vi "myRIO_BRig_FPGA_v3,1__PortC.vi"() -> ()   [LabVIEW 2014]
uses:
  <vilib>/rvi/FXPMathLib/FxpDiv/subVIs/nifxpmath_Div_SimConfig.ctl
  <vilib>/rvi/FXPMathLib/FxpSinAndCos/subVIs/nifxpmath_SinAndCos_SimConfig.ctl
  <vilib>/rvi/FXPMathLib/FxpDiv/simVIs/DllFxpDivTemp_sub.vi
  <vilib>/rvi/FXPMathLib/FxpSinAndCos/simVIs/DllFxpSinAndCosTemp_sub.vi
  <vilib>/rvi/Emulation/niFpgaGetClockAttributes.vi
  <vilib>/rvi/Emulation/niFpgaSctlEmulationGetInTimedLoop.vi
  <vilib>/rvi/Emulation/niFpgaEmulationReportErrorSimple.vi
  <vilib>/rvi/eio/common/nirviEmuTemplateMethod_errors.vi
  <vilib>/rvi/Emulation/niFpgaCriticalErrorInLSC.vi
  <vilib>/rvi/FXPMathLib/FxpDiv/XNode/nifxpmath_Div.xnode
  <vilib>/rvi/FXPMathLib/FxpMul/XNode/nifxpmath_Multiplier.xnode
  <vilib>/rvi/FXPMathLib/FxpSinAndCos/XNode/nifxpmath_SinAndCos.xnode
  <vilib>/rvi/FXPMathLib/FxpSub/XNode/nifxpmath_Sub.xnode
  <vilib>/eio/EIONode/EIONode.xnode
  <vilib>/rvi/FXPMathLib/sim/FxpSim.dll
panel:
  in  "AO0":i16
  in  "f_time_select":u32=173
  in  "laser_Nvalley":u32=100
  in  "laser_Npeak":u32=100
  in  "laserledMTrig":bool
  in  "tCycle_laser_wro":u32=100
  in  "tDelay_laser_wro":u32
  in  "tCycle_laser_rew":u32=100
  in  "tDelay_laser_rew":u32
  in  "laserResponse_reward_LED":bool
  in  "laserResponse_wrong_LED":bool
  out "SelectWrong":bool
  out "SelectReward":bool
  in  "laserResponse_wrong":bool
  in  "laserResponse_reward":bool
  in  "Left(F)_or_Right(T)":bool
  in  "ignoreWrong":bool
  in  "SelectionState":bool
  in  "laserMTrig":bool
  in  "FPGA_Stop":bool
  in  "audioTrigger_L":bool
  in  "audioTrigger_R":bool
  in  "audioFreq_L_Hz":u16=1000 min=1000 max=14000 step=1000
  in  "audioAmp_L":u16=1 min=1 max=32767 step=1
  in  "audioFreq_R_Hz":u16=1000 min=1000 max=14000 step=1000
  in  "audioAmp_R":u16=1 min=1 max=32767 step=1
  in  "A3_SL":bool
  in  "A1_SR":bool
  in  "Counts_Reset":bool
  out "A4_LickR":u32
  out "A2_LickL":u32
  in  "A6_Act":bool
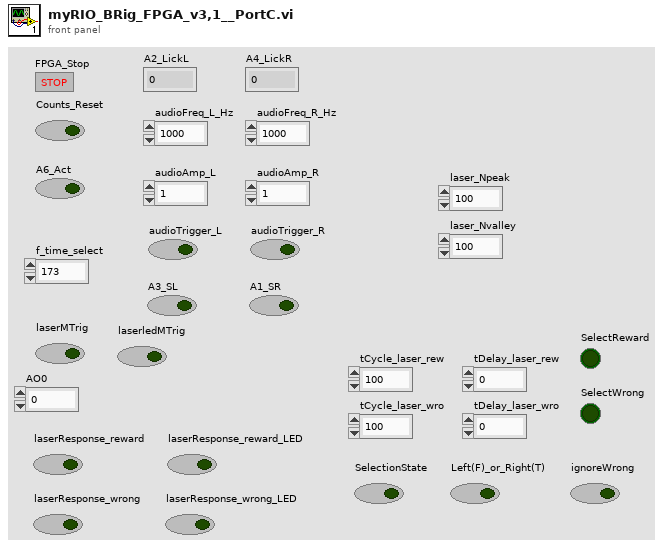
[diagram p1: front panel]
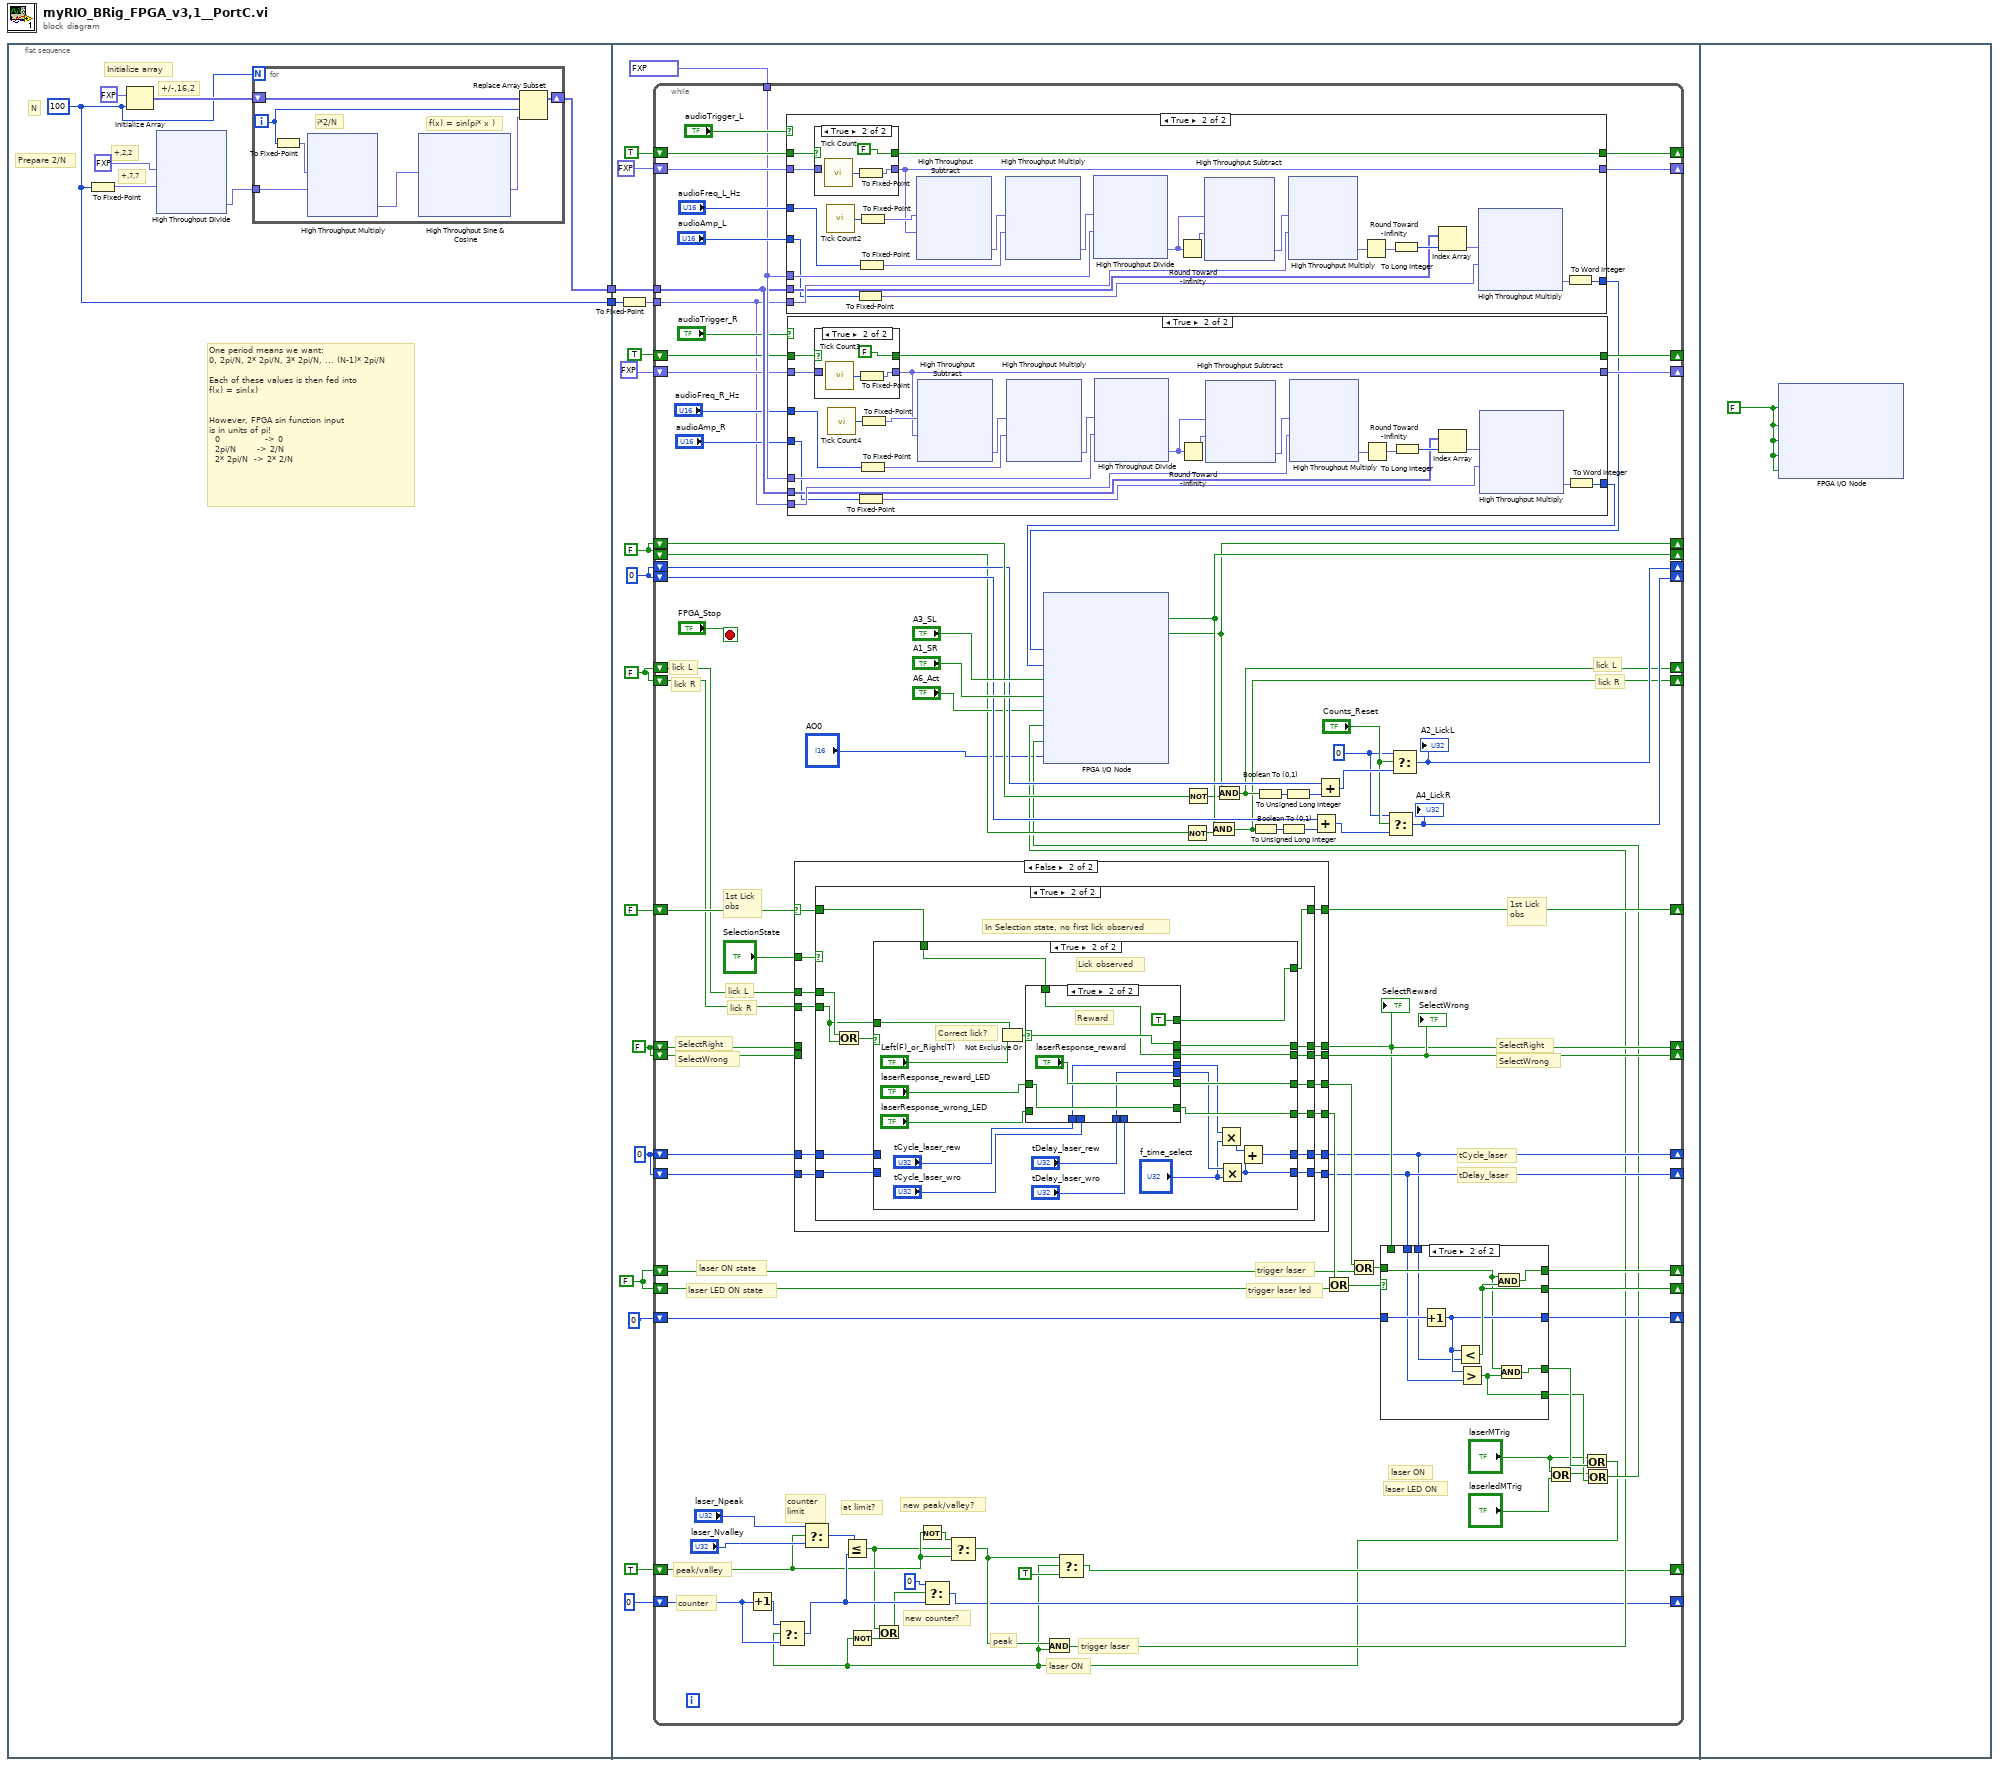
[diagram p0: block diagram]
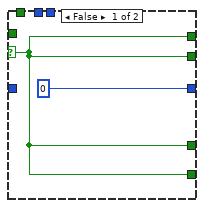
[diagram p2: hidden frame]
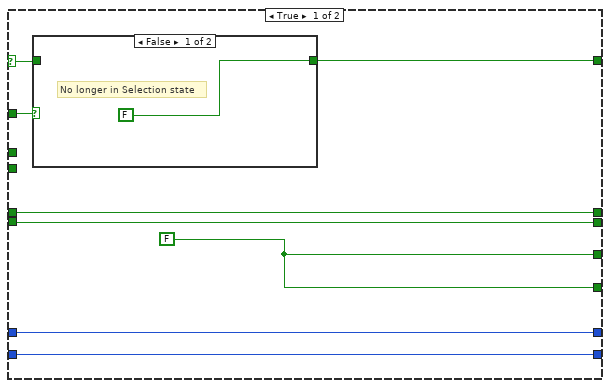
[diagram p3: hidden frame]
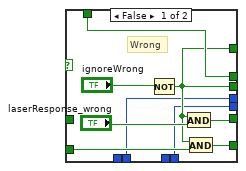
[diagram p7: hidden frame]
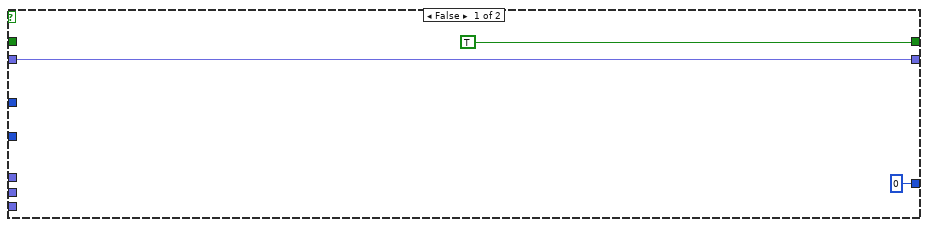
[diagram p8: hidden frame]
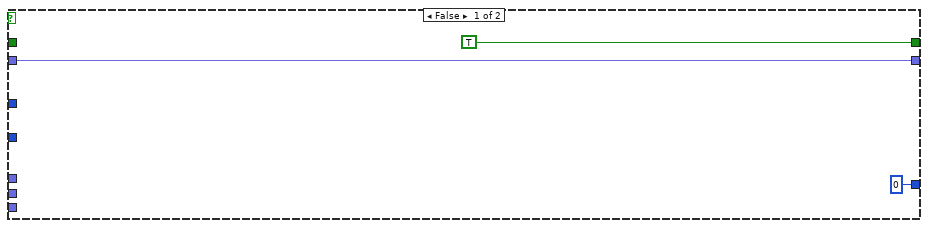
[diagram p10: hidden frame]
diagram:
  n1 = flat-sequence {
    tunnel: [w4] -> w2
    tunnel: [w3] -> w1
    tunnel: w2 -> [w86]
    tunnel: w1 -> [w88]
    frame #0 {
      w3 = 100 ("dimension size")
      # "N"
      # "+,7,7"
      # "+,2,2"
      # "+/-,16,2"
      # "Prepare 2/N"
      # "One period means we want:\n0, 2pi/N, 2* 2pi/N, 3* 2pi/N, ... (N-1)* 2pi/N\n\nEach of these values is then fed into\nf(x) = sin(x)\n\n\nHowever, FPGA sin function input\nis in units of pi!\n  0               -> 0\n  2pi/N       -> 2/N\n  2* 2pi/N  -> 2* 2/N"
      # "Initialize array"
      n2 = To Fixed-Point(number=w3) -> (fixed-point=w6:fxp<+,7,7>)  [unwired: 1 in]
      n3 = Initialize Array(fxp<+/-,16,2> 0.0 ("element"), w3) -> (w9:fxp<+/-,16,2>[])
      n4 = xnode "High Throughput Divide"("x"=fxp<+,2,2> 2.0, "y"=w6) -> ("x/y"=w5:fxp<+,27,0>)
      n5 = for {
        N: w3 -> [_]
        shift-right: [w42] -> w4
        shift-left: w9 -> [w43]
        tunnel: w5 -> [w38]
        i -> [w41]
        # "f(x) = sin(pi* x )"
        # "i*2/N"
        n6 = To Fixed-Point(number=w41) -> (fixed-point=w39:fxp<+,7,7>)  [unwired: 1 in]
        n7 = xnode ("High Throughput Multiply")("x"=w39, "y"=w38) -> ("x*y"=w37:fxp<+,34,7>)
        n8 = xnode "High Throughput Sine & Cosine"("x (pi)"=w37) -> ("sin(x)"=w40:fxp<+/-,16,2>)  [unwired: 1 out]
        n9 = Replace Array Subset(array=w43, new element=w40, index=w41) -> (w42:fxp<+/-,16,2>[])
      }
    }
    frame #1 {
      w76 = u32 0
      w78 = FALSE
      w77 = FALSE
      w81 = FALSE
      w82 = FALSE
      w83 = u32 0
      n10 = To Fixed-Point(number=w88) -> (fixed-point=w87:fxp<+,7,7>)  [unwired: 1 in]
      n11 = while {
        shift-right: [w176] -> _
        shift-left: TRUE -> [w180]
        shift-right: [w175] -> _
        shift-left: fxp<+,32,32> 0.0 -> [w179]
        tunnel: fxp<+,17,26> 40000000.0 -> [w174]
        tunnel: w87 -> [w167]
        tunnel: w86 -> [w173]
        shift-right: [w166] -> _
        shift-left: TRUE -> [w172]
        shift-right: [w165] -> _
        shift-left: fxp<+,32,32> 0.0 -> [w171]
        shift-right: [w142] -> _
        shift-left: w83 -> [w154]
        shift-right: [w145] -> _
        shift-left: w83 -> [w158]
        shift-right: [w146] -> _
        shift-left: w82 -> [w149]
        shift-right: [w143] -> _
        shift-left: w82 -> [w155]
        shift-right: [w140] -> _
        shift-left: FALSE -> [w139]
        shift-right: [w138] -> _
        shift-left: w81 -> [w136]
        shift-right: [w137] -> _
        shift-left: w81 -> [w135]
        shift-right: [w125] -> _
        shift-left: w77 -> [w127]
        shift-right: [w133] -> _
        shift-left: u32 0 -> [w134]
        shift-right: [w119] -> _
        shift-left: w78 -> [w131]
        shift-right: [w132] -> _
        shift-left: w78 -> [w130]
        shift-right: [w126] -> _
        shift-left: w77 -> [w123]
        shift-right: [w115] -> _
        shift-left: w76 -> [w118]
        shift-right: [w116] -> _
        shift-left: w76 -> [w117]
        shift-right: [w97] -> _
        shift-left: u32 0 -> [w109]
        shift-right: [w98] -> _
        shift-left: TRUE -> [w101]
        stop <- "FPGA_Stop" stop-if-true
        w151 = u32 0
        # "trigger laser"
        # "peak"
        # "laser ON"
        # "new peak/valley?"
        # "counter"
        # "peak/valley"
        # "new counter?"
        # "at limit?"
        # "counter\nlimit"
        # "tDelay_laser"
        # "tCycle_laser"
        # "laser LED ON"
        # "laser ON"
        # "laser LED ON state"
        # "laser ON state"
        # "SelectWrong"
        # "SelectRight"
        # "SelectWrong"
        # "SelectRight"
        # "lick R"
        # "lick L"
        # "1st Lick\nobs"
        # "1st Lick\nobs"
        # "lick R"
        # "lick L"
        # "lick R"
        # "lick L"
        # "trigger laser led"
        # "trigger laser"
        n12 = Increment(x=w109) -> (x+1=w107:u32)
        n13 = case shown="True" "audioTrigger_L" {
          tunnel: w180 -> [_ w358]
          tunnel: w179 -> [w334 w357]
          tunnel: "audioFreq_L_Hz" -> [_ w354]
          tunnel: w174 -> [_ w351]
          tunnel: [w334 w335] -> w175
          tunnel: [TRUE w348] -> w176
          tunnel: w167 -> [_ w347]
          tunnel: w173 -> [_ w342]
          tunnel: "audioAmp_L" -> [_ w340]
          tunnel: [i16 0 w337] -> w161
          frame False {
          }
          frame True {
            n14 = case shown="True" w358 {
              selector: w358 -> [w387 _]
              tunnel: [w387 FALSE] -> w348
              tunnel: w357 -> [w386 _]
              tunnel: [w386 w388] -> w335
              frame False {
              }
              frame True {
                n15 = call "Tick Count"() -> ("Tick Count(Ticks)"=w390:u32)
                n16 = To Fixed-Point(number=w390) -> (fixed-point=w388:fxp<+,32,32>)  [unwired: 1 in]
              }
            }
            n17 = call "Tick Count2"() -> ("Tick Count(Ticks)"=w356:u32)
            n18 = To Fixed-Point(number=w340) -> (fixed-point=w339:fxp<+,15,15>)  [unwired: 1 in]
            n19 = To Fixed-Point(number=w354) -> (fixed-point=w353:fxp<+,14,14>)  [unwired: 1 in]
            n20 = To Fixed-Point(number=w356) -> (fixed-point=w336:fxp<+,32,32>)  [unwired: 1 in]
            n21 = xnode "High Throughput Subtract"("x"=w336, "y"=w335) -> ("x-y"=w355:fxp<+,32,32>)
            n22 = xnode ("High Throughput Multiply")("x"=w355, "y"=w353) -> ("x*y"=w352:fxp<+,46,46>)
            n23 = xnode "High Throughput Divide"("x"=w352, "y"=w351) -> ("x/y"=w350:fxp<+,34,21>)
            n24 = Round Toward -Infinity(1:w350) -> (0:w349:fxp<+,21,21>)
            n25 = xnode "High Throughput Subtract"("x"=w350, "y"=w349) -> ("x-y"=w346:fxp<+,14,1>)
            n26 = xnode ("High Throughput Multiply")("x"=w346, "y"=w347) -> ("x*y"=w343:fxp<+,21,8>)
            n27 = Round Toward -Infinity(1:w343) -> (0:w345:fxp<+,8,8>)
            n28 = To Long Integer(number=w345) -> (32bit integer=w344:i32)
            n29 = Index Array(array=w342, index=w344) -> (element=w341:fxp<+/-,16,2>)
            n30 = xnode ("High Throughput Multiply")("x"=w341, "y"=w339) -> ("x*y"=w338:fxp<+/-,31,17>)
            n31 = To Word Integer(number=w338) -> (16bit integer=w337:i16)
          }
        }
        n32 = case shown="True" "audioTrigger_R" {
          tunnel: w172 -> [_ w299]
          tunnel: w171 -> [w275 w298]
          tunnel: "audioFreq_R_Hz" -> [_ w295]
          tunnel: w174 -> [_ w292]
          tunnel: [w275 w276] -> w165
          tunnel: [TRUE w289] -> w166
          tunnel: w167 -> [_ w288]
          tunnel: w173 -> [_ w283]
          tunnel: "audioAmp_R" -> [_ w281]
          tunnel: [i16 0 w278] -> w162
          frame False {
          }
          frame True {
            n33 = case shown="True" w299 {
              selector: w299 -> [w328 _]
              tunnel: [w328 FALSE] -> w289
              tunnel: w298 -> [w327 _]
              tunnel: [w327 w329] -> w276
              frame False {
              }
              frame True {
                n34 = call "Tick Count3"() -> ("Tick Count(Ticks)"=w331:u32)
                n35 = To Fixed-Point(number=w331) -> (fixed-point=w329:fxp<+,32,32>)  [unwired: 1 in]
              }
            }
            n36 = call "Tick Count4"() -> ("Tick Count(Ticks)"=w297:u32)
            n37 = To Fixed-Point(number=w281) -> (fixed-point=w280:fxp<+,15,15>)  [unwired: 1 in]
            n38 = To Fixed-Point(number=w295) -> (fixed-point=w294:fxp<+,14,14>)  [unwired: 1 in]
            n39 = To Fixed-Point(number=w297) -> (fixed-point=w277:fxp<+,32,32>)  [unwired: 1 in]
            n40 = xnode "High Throughput Subtract"("x"=w277, "y"=w276) -> ("x-y"=w296:fxp<+,32,32>)
            n41 = xnode ("High Throughput Multiply")("x"=w296, "y"=w294) -> ("x*y"=w293:fxp<+,46,46>)
            n42 = xnode "High Throughput Divide"("x"=w293, "y"=w292) -> ("x/y"=w291:fxp<+,34,21>)
            n43 = Round Toward -Infinity(1:w291) -> (0:w290:fxp<+,21,21>)
            n44 = xnode "High Throughput Subtract"("x"=w291, "y"=w290) -> ("x-y"=w287:fxp<+,14,1>)
            n45 = xnode ("High Throughput Multiply")("x"=w287, "y"=w288) -> ("x*y"=w284:fxp<+,21,8>)
            n46 = Round Toward -Infinity(1:w284) -> (0:w286:fxp<+,8,8>)
            n47 = To Long Integer(number=w286) -> (32bit integer=w285:i32)
            n48 = Index Array(array=w283, index=w285) -> (element=w282:fxp<+/-,16,2>)
            n49 = xnode ("High Throughput Multiply")("x"=w282, "y"=w280) -> ("x*y"=w279:fxp<+/-,31,17>)
            n50 = To Word Integer(number=w279) -> (16bit integer=w278:i16)
          }
        }
        n51 = case shown="False" w139 {
          selector: w139 -> [w199 w214]
          tunnel: "SelectionState" -> [w201 w216]
          tunnel: [w200 w215] -> w140
          tunnel: w136 -> [_ w213]
          tunnel: w135 -> [_ w212]
          tunnel: [w198 w211] -> w124
          tunnel: [w196 w210] -> w119
          tunnel: [w197 w209] -> w132
          tunnel: w131 -> [w196 _]
          tunnel: w130 -> [w197 _]
          tunnel: [w198 w208] -> w128
          tunnel: [w195 w207] -> w115
          tunnel: [w194 w206] -> w116
          tunnel: w118 -> [w195 w205]
          tunnel: w117 -> [w194 w204]
          frame True {
            w198 = FALSE
            n52 = case shown="False" w201 {
              tunnel: [FALSE w203] -> w200
              tunnel: w199 -> [_ w203]
              frame False {
                # "No longer in Selection state"
              }
              frame True {
                # "Already observed first lick, no other action"
              }
            }
          }
          frame False {
            n53 = case shown="True" w216 {
              tunnel: [w219 w229] -> w215
              tunnel: w214 -> [w219 w225]
              tunnel: w213 -> [_ w231]
              tunnel: w212 -> [_ w230]
              tunnel: [w219 w228] -> w211
              tunnel: [w219 w227] -> w210
              tunnel: [w219 w226] -> w209
              tunnel: [w219 w224] -> w208
              tunnel: [w218 w223] -> w207
              tunnel: [w217 w222] -> w206
              tunnel: w205 -> [w218 w221]
              tunnel: w204 -> [w217 w220]
              frame False {
                # "Not in Selection state"
              }
              frame True {
                # "In Selection state, no first lick observed"
                n54 = Or(x=w231, y=w230) -> (x .or. y?=w232:bool)
                n55 = case shown="True" w232 {
                  tunnel: w230 -> [_ w255]
                  tunnel: [w235 w248] -> w229
                  tunnel: [w235 w253] -> w228
                  tunnel: [w235 w252] -> w227
                  tunnel: [w235 w251] -> w226
                  tunnel: w225 -> [w235 w250]
                  tunnel: [w235 w249] -> w224
                  tunnel: [w234 w237] -> w223
                  tunnel: [w233 w236] -> w222
                  tunnel: w221 -> [w234 _]
                  tunnel: w220 -> [w233 _]
                  frame False {
                  }
                  frame True {
                    # "Correct lick?"
                    # "Lick observed"
                    n56 = Not Exclusive Or(1:"Left(F)_or_Right(T)", 2:w255) -> (0:w254:bool)
                    n57 = case shown="True" w254 {
                      selector: w254 -> [_ w271]
                      tunnel: [w262 "laserResponse_reward"] -> w253
                      tunnel: [w260 w267] -> w251
                      tunnel: [w264 w271] -> w252
                      tunnel: w250 -> [w264 w267]
                      tunnel: [w261 w269] -> w249
                      tunnel: [w260 TRUE] -> w248
                      tunnel: "laserResponse_reward_LED" -> [_ w269]
                      tunnel: "laserResponse_wrong_LED" -> [w259 _]
                      tunnel: "tCycle_laser_rew" -> [_ w266]
                      tunnel: "tCycle_laser_wro" -> [w257 _]
                      tunnel: "tDelay_laser_rew" -> [_ w268]
                      tunnel: "tDelay_laser_wro" -> [w258 _]
                      tunnel: [w258 w268] -> w240
                      tunnel: [w257 w266] -> w239
                      frame False {
                        # "Wrong"
                        n58 = Not(x="ignoreWrong") -> (.not. x?=w260:bool)
                        n59 = And(x=w260, y="laserResponse_wrong") -> (x .and. y?=w262:bool)
                        n60 = And(x=w260, y=w259) -> (x .and. y?=w261:bool)
                      }
                      frame True {
                        # "Reward"
                      }
                    }
                    n61 = Multiply(x=w239, y="f_time_select") -> (x*y=w241:u32)
                    n62 = Multiply(x=w240, y="f_time_select") -> (x*y=w236:u32)
                    n63 = Add(x=w241, y=w236) -> (x+y=w237:u32)
                  }
                }
              }
            }
          }
        }
        "SelectWrong" <- w132
        "SelectReward" <- w119
        n64 = Select(t="laser_Npeak", s=w101, f="laser_Nvalley") -> (s? t:f=w111:u32)
        n65 = Not(x=w101) -> (.not. x?=w102:bool)
        n66 = Not(x=w149) -> (.not. x?=w148:bool)
        n67 = Not(x=w155) -> (.not. x?=w144:bool)
        n68 = Or(x=w128, y=w127) -> (x .or. y?=w129:bool)
        n69 = Or(x=w124, y=w123) -> (x .or. y?=w122:bool)
        n70 = case shown="True" w129 {
          selector: w129 -> [w183 _]
          tunnel: w134 -> [_ w193]
          tunnel: [u32 0 w190] -> w133
          tunnel: [w183 w191] -> w125
          tunnel: [w183 w192] -> w126
          tunnel: w122 -> [_ w189]
          tunnel: [w183 w188] -> w120
          tunnel: [w183 w187] -> w121
          tunnel: w119 -> [_ _]
          tunnel: w116 -> [_ w186]
          tunnel: w115 -> [_ w185]
          frame False {
          }
          frame True {
            n71 = Increment(x=w193) -> (x+1=w190:u32)
            n72 = Less?(x=w190, y=w185) -> (x < y?=w191:bool)
            n73 = Greater?(x=w190, y=w186) -> (0:w188:bool)
            n74 = And(x=w189, y=w191) -> (x .and. y?=w192:bool)
            n75 = And(x=w189, y=w188) -> (x .and. y?=w187:bool)
          }
        }
        n76 = Or(x="laserMTrig", y="laserledMTrig") -> (x .or. y?=w113:bool)
        n77 = Or(x="laserMTrig", y=w121) -> (x .or. y?=w95:bool)
        n78 = Select(t=w107, s=w95, f=w109) -> (s? t:f=w106:u32)
        n79 = Less Or Equal?(x=w111, y=w106) -> (x <= y?=w94:bool)
        n80 = Not(x=w95) -> (.not. x?=w96:bool)
        n81 = Or(x=w94, y=w96) -> (x .or. y?=w93:bool)
        n82 = Select(t=u32 0, s=w93, f=w106) -> (s? t:f=w97:u32)
        n83 = Select(t=w102, s=w94, f=w101) -> (s? t:f=w100:bool)
        n84 = And(x=w100, y=w95) -> (x .and. y?=w103:bool)
        n85 = Select(t=w100, s=w95, f=TRUE) -> (s? t:f=w98:bool)
        n86 = Or(x=w113, y=w120) -> (x .or. y?=w108:bool)
        n87 = xnode "FPGA I/O Node"("AudioOut/Left"=w161, "AudioOut/Right"=w162, "ConnectorC/DIO3"="A3_SL", "ConnectorC/DIO1"="A1_SR", "ConnectorC/DIO6"="A6_Act", "ConnectorC/DIO0"=w103, "ConnectorC/DIO7"=w108, "ConnectorC/AO0"="AO0") -> ("ConnectorC/DIO4"=w146:bool, "ConnectorC/DIO2"=w143:bool)  [unwired: 10 in, 10 out]
        n88 = And(x=w146, y=w148) -> (x .and. y?=w137:bool)
        n89 = And(x=w143, y=w144) -> (x .and. y?=w138:bool)
        n90 = Boolean To (0,1)(Boolean=w137) -> (0, 1=w160:i16)
        n91 = Boolean To (0,1)(Boolean=w138) -> (0, 1=w157:i16)
        n92 = To Unsigned Long Integer(number=w160) -> (unsigned 32bit integer=w159:u32)
        n93 = To Unsigned Long Integer(number=w157) -> (unsigned 32bit integer=w156:u32)
        n94 = Add(x=w158, y=w159) -> (x+y=w147:u32)
        n95 = Add(x=w154, y=w156) -> (x+y=w153:u32)
        n96 = Select(t=w151, s="Counts_Reset", f=w147) -> (s? t:f=w145:u32)
        "A4_LickR" <- w145
        n97 = Select(t=w151, s="Counts_Reset", f=w153) -> (s? t:f=w142:u32)
        "A2_LickL" <- w142
      }
    }
    frame #2 {
      w391 = FALSE ("ConnectorA/DIO3")
      n98 = xnode "FPGA I/O Node"("ConnectorC/DIO3"=w391, "ConnectorC/DIO1"=w391, "ConnectorC/DIO0"=w391, "ConnectorC/DIO6"=w391, "ConnectorC/DIO7"=w391) -> ()  [unwired: 5 in, 5 out]
    }
  }
